vi "Configure Socket Port Number.vi"(8 "error in (no error)":errorcluster, 9 "Port Number (0)":i32, 10 "Channel (1)":i32=1, 11 "VISA resource name":refnum<visa-resource-name>) -> (0 "error out":errorcluster, 3 "VISA resource name out":refnum<visa-resource-name>)   [LabVIEW 2020, in "Rohde&Schwarz CMXP Base.lvlib"]
doc: "Sets the data port number for direct socket communication.\n\nAttribute:\nRSCMXPBASE_ATTR_SET_DIRECT_PORT_NUMBER\n\nRemote-control command:\nSYSTem:COMMunicate:SOCKet<i>:PORT"
uses:
  <instrlib>/Rohde&Schwarz CMXP Base/Rohde&Schwarz CMXP Base.lvlib
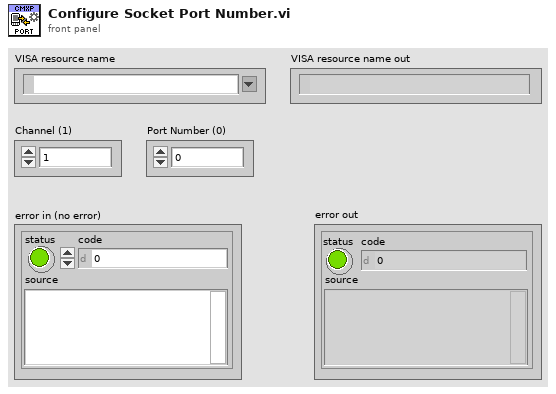
[diagram p1: front panel]
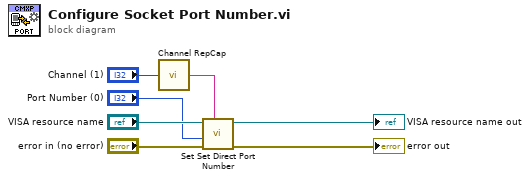
[diagram p0: block diagram]
diagram:
  n1 = call <instrlib>:"Channel RepCap.vi"("Channel In"="Channel (1)") -> ("Channel Out"=w2:string)  [unwired: 1 out]
  n2 = call "Set Set Direct Port Number"("Repeated Capabilities"=w2, "error in (no error)"="error in (no error)", "Set Direct Port Number (0)"="Port Number (0)", "instrument handle"="VISA resource name") -> ("error out"=→"error out":errorcluster, "instrument handle out"=→"VISA resource name out":refnum<visa-resource-name>)  [unwired: 6 in]
